vi "Array to Multi Ch Waveforms.vi"(8 "channel names":string[](array[string]), 10 "dt":dbl, 11 "array":dbl[](array[numeric])) -> (3 "waveforms":waveform(dbl)[](array[waveform]))   [LabVIEW 2021]
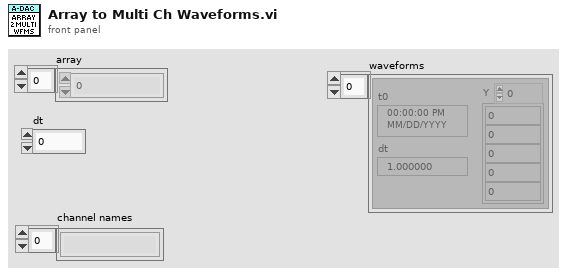
[diagram p1: front panel]
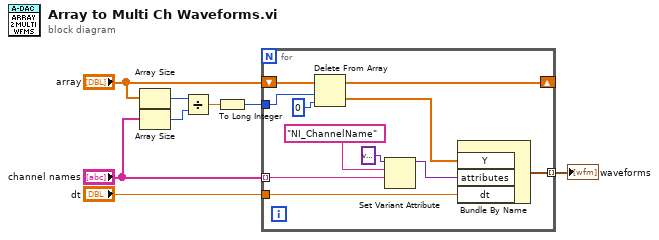
[diagram p0: block diagram]
diagram:
  n1 = Array Size(array="array") -> (size(s)=w8:i32)
  n2 = Array Size(array="channel names") -> (size(s)=w7:i32)
  n3 = Divide(x=w8, y=w7) -> (x/y=w5:dbl)
  n4 = To Long Integer(number=w5) -> (32bit integer=w4:i32)
  n5 = for {
    shift-right: [w18] -> _
    shift-left: "array" -> [w19]
    tunnel: w4 -> [w16]
    tunnel: "channel names" -> [w14] mode=indexing
    tunnel: "dt" -> [w9]
    tunnel: [w12] -> w1 mode=indexing
    n6 = Delete From Array(array=w19, length=w16, index=0) -> (deleted portion=w10:dbl[], array with subset deleted=w18:dbl[])
    n7 = Set Variant Attribute(Variant=variant ("variant"), name="NI_ChannelName", value=w14) -> (Variant out=w15:variant)  [unwired: 1 in, 2 out]
    n8 = Bundle By Name("Y"=w10, "attributes"=w15, "dt"=w9) -> (w12:waveform(dbl))  [unwired: 1 in]
  }
  "waveforms" <- w1
